vi "Name Assert Display.vi"(8 "error in (no error)":errorcluster, 11 "Assert Display in":refnum<class "Assert Display.lvclass">) -> (0 "error out":errorcluster, 2 "Build?":bool, 3 "Assert Display out":refnum<class "Assert Display.lvclass">)   [LabVIEW 2016, in "Assert API Components.lvlib" / "Assert Display.lvlib" / "Assert Display.lvclass"]
uses:
  Assert Display.lvclass
  Assert Display.lvclass/Assert Display.ctl
panel:
  in  "OK":bool
  in  "Name":string
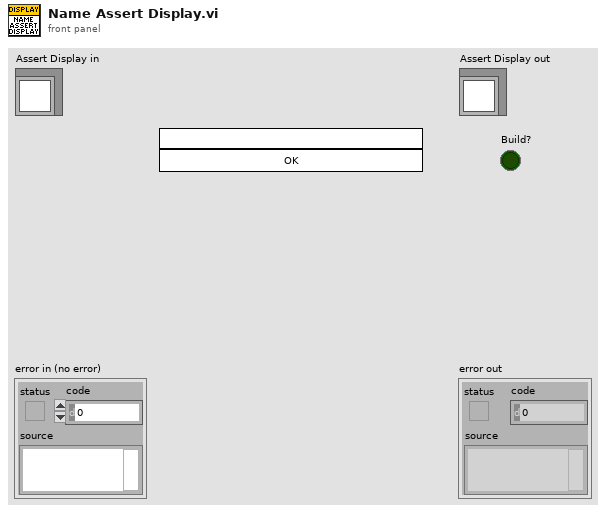
[diagram p1: front panel]
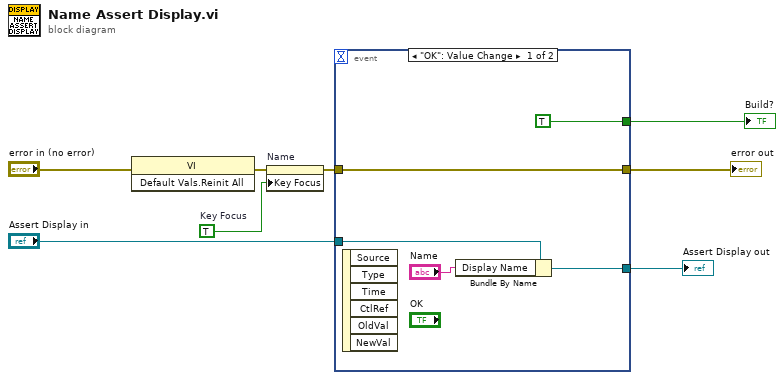
[diagram p0: block diagram]
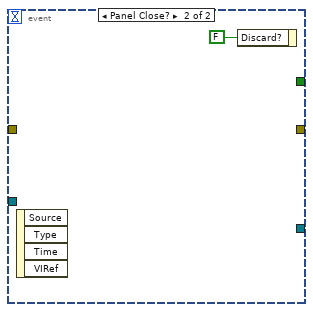
[diagram p2: hidden frame]
diagram:
  w4 = TRUE  # Key Focus
  n1 = invoke class="VI" method="Default Vals.Reinit All"(error in="error in (no error)") -> (error out=w5:errorcluster)  [unwired: 2 in, 2 out]
  n2 = property on="Name" class="Str"(error in=w5, "Key Focus"=w4) -> (error out=w3:errorcluster)  [unwired: 1 in, 1 out]
  n3 = event shown="[0] \"OK\": Value Change" {
    selector: _ -> [_ _]
    dyn-events: _ -> [_ _]
    timeout: _ -> [_ _]
    tunnel: "Assert Display in" -> [w13 _]
    tunnel: [w12 _] -> w6
    tunnel: w3 -> [w10 _]
    tunnel: [w10 _] -> w2
    tunnel: [TRUE _] -> w1
    event "OK": Value Change {
      n4 = event-data() -> ()  [unwired: 1 in, 6 out]
      n5 = Bundle By Name(cluster=w13, "Display Name"="Name") -> (w12:refnum<class "Assert Display.lvclass">)
    }
    event Panel Close? {
      n6 = event-data() -> ()  [unwired: 1 in, 4 out]
      n7 = event-data("Discard?"=FALSE) -> ()  [unwired: 1 in, 1 out]
    }
  }
  "error out" <- w2
  "Assert Display out" <- w6
  "Build?" <- w1
